vi "Initialize-user-events.vi"(8 "error in (no error)":errorcluster, 11 "ModComm in":T1) -> (0 "error out":errorcluster, 3 "ModComm out":T1)   [LabVIEW 2013, in "SLMServer.lvlib" / "SLMServer.lvclass"]
uses:
  SLMServer.lvclass
  Object-reference.ctl
  SLMServer.lvclass/SLMServer.ctl
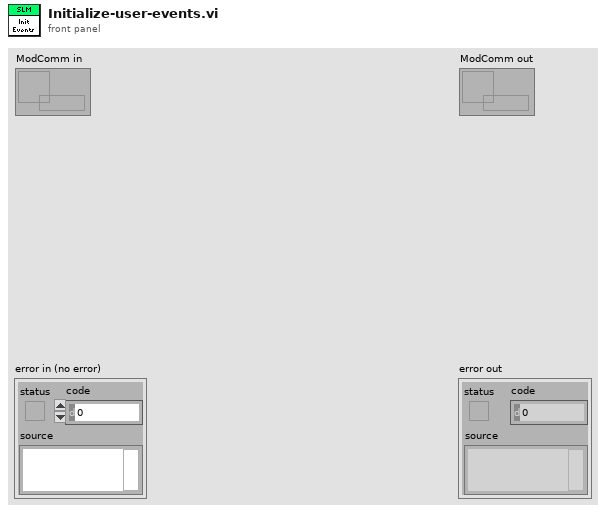
[diagram p1: front panel]
types:
  T1 = typedef "SLMServer.lvlib/SLMServer.lvclass/Object-reference.ctl" = refnum<data-value>
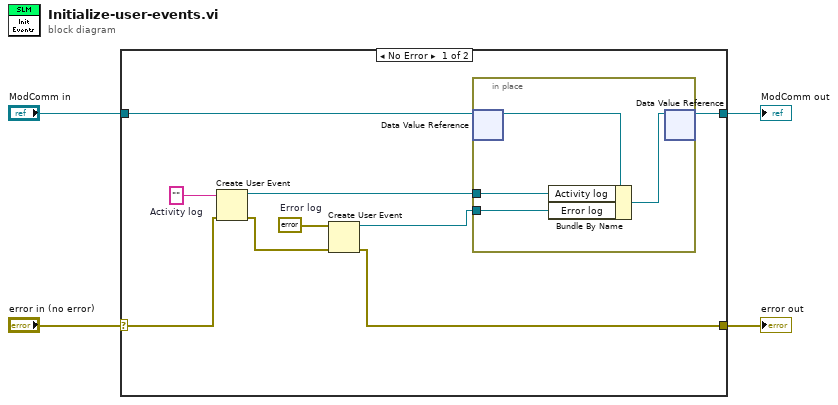
[diagram p0: block diagram]
diagram:
  n1 = case shown="No Error" "error in (no error)" {
    selector: "error in (no error)" -> [w10 w19]
    tunnel: [w6 w19] -> w3
    tunnel: [w5 w18] -> w1
    tunnel: "ModComm in" -> [w9 w18]
    frame No Error {
      w12 = errorcluster {"status"=FALSE, "code"=0, "source"=""}  # Error log
      w13 = ""  # Activity log
      n2 = Create User Event(user event datatype=w13, error in=w10) -> (user event=w8:refnum<user-event>, error out=w11:errorcluster)
      n3 = Create User Event(user event datatype=w12, error in=w11) -> (user event=w7:refnum<user-event>, error out=w6:errorcluster)
      n4 = in-place {
        in-place-border: w8 -> [w16]
        in-place-border: w7 -> [w15]
        n5 = in-place-dvr #1(w9) -> (w17:refnum<class "SLMServer.lvclass">)  [unwired: 1 out]
        n6 = Bundle By Name(cluster=w17, "Activity log"=w16, "Error log"=w15) -> (w14:refnum<class "SLMServer.lvclass">)
        n7 = in-place-dvr #1(w14) -> (w5:T1)  [unwired: 1 out]
      }
    }
    frame Error {
    }
  }
  "error out" <- w3
  "ModComm out" <- w1
